vi "修改-微调探头测量值-30.vi"(8 "VI引用句柄":refnum<vi>, 10 "探头地址":i32, 11 "VISA资源名称":refnum<visa-resource-name>) -> (0 "结果":T1)   [LabVIEW 2017]
panel:
  in  "取消按钮":bool
  in  "确定按钮":bool
  in  "微调方向":enum8{"减小", "增大"}(ring)
  in  "微调值 uSv/h":sgl=0.03 min=0 max=655.36 format="%#.2f"
  out "提示语":string
  # "提示：微调值直接修改探头硬件参数，\n软件中无修改记录，请谨慎修改"
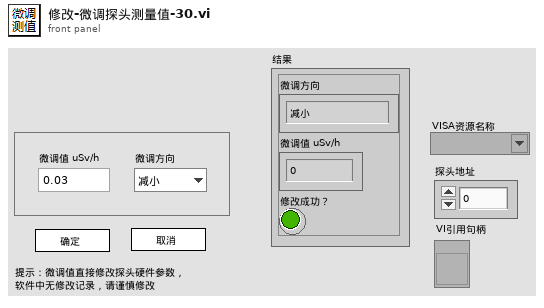
[diagram p1: front panel]
types:
  T1 = cluster{"微调方向":enum8{"减小", "增大"}, "微调值 uSv/h":sgl, "修改成功？":bool}
  T2 = enum32{"Invalid", "Standard", "Closed", "Hidden", "Minimized", "Maximized"}
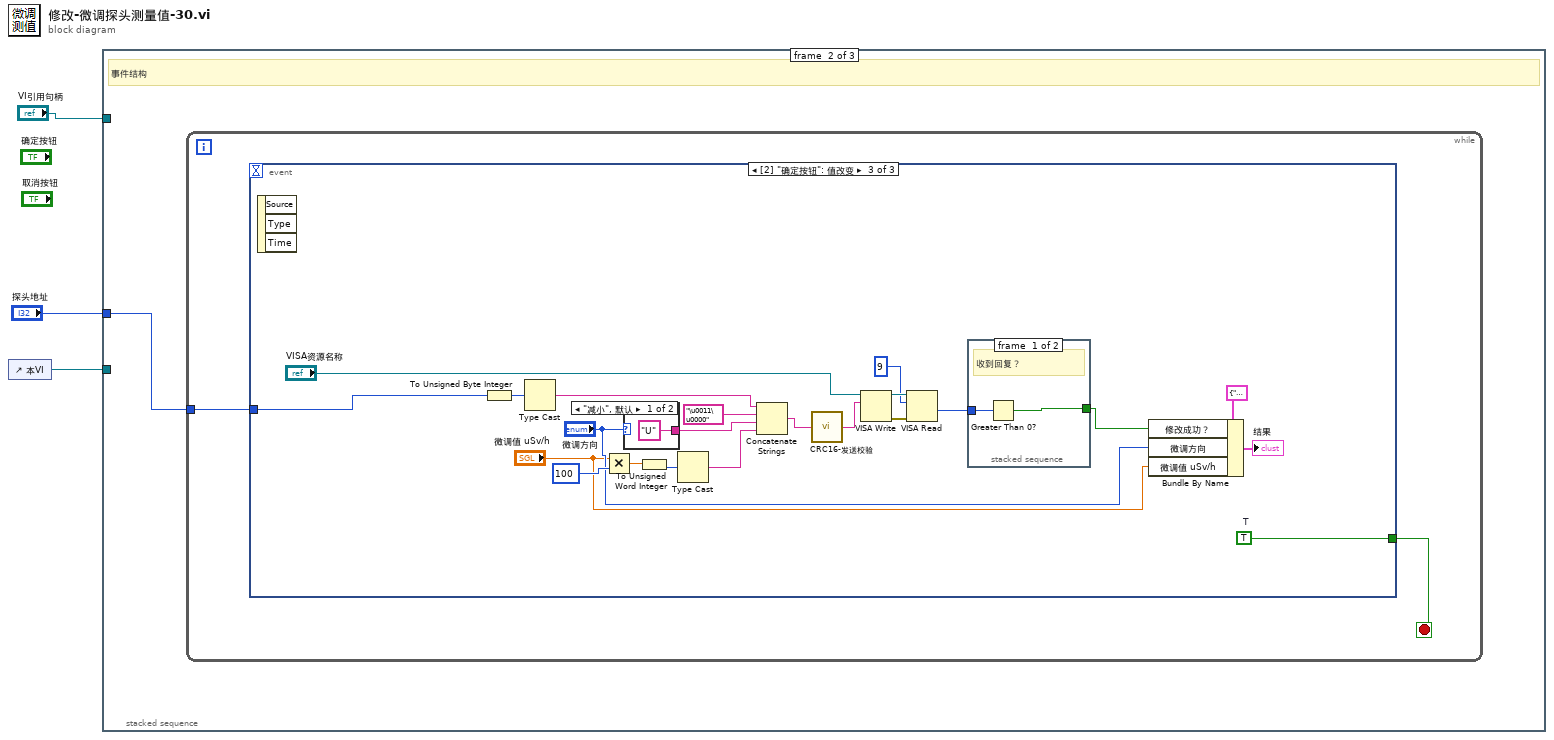
[diagram p0: block diagram]
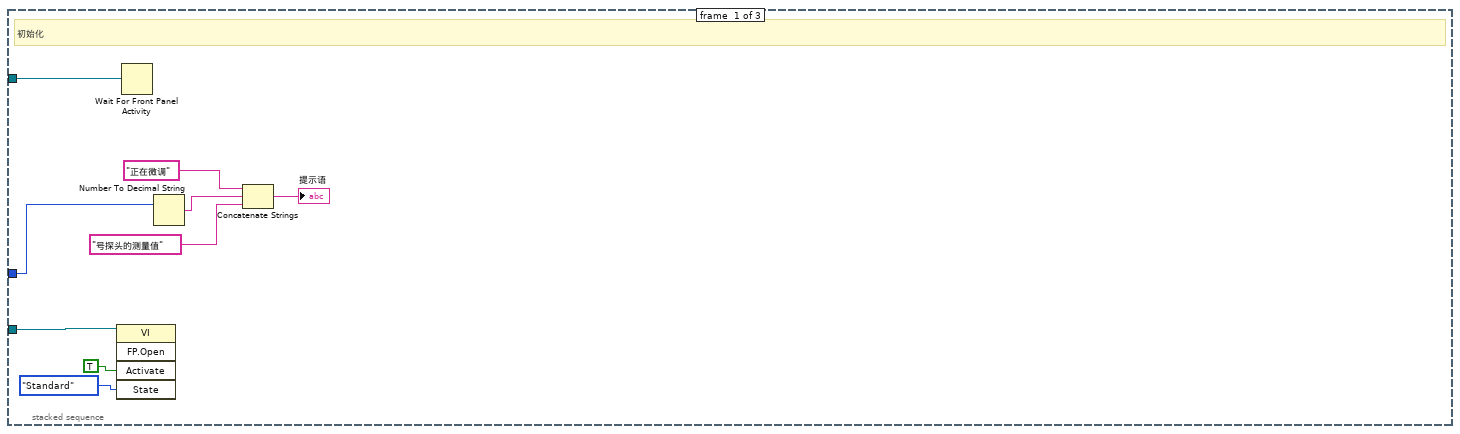
[diagram p2: hidden frame]
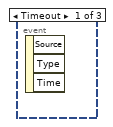
[diagram p3: hidden frame]
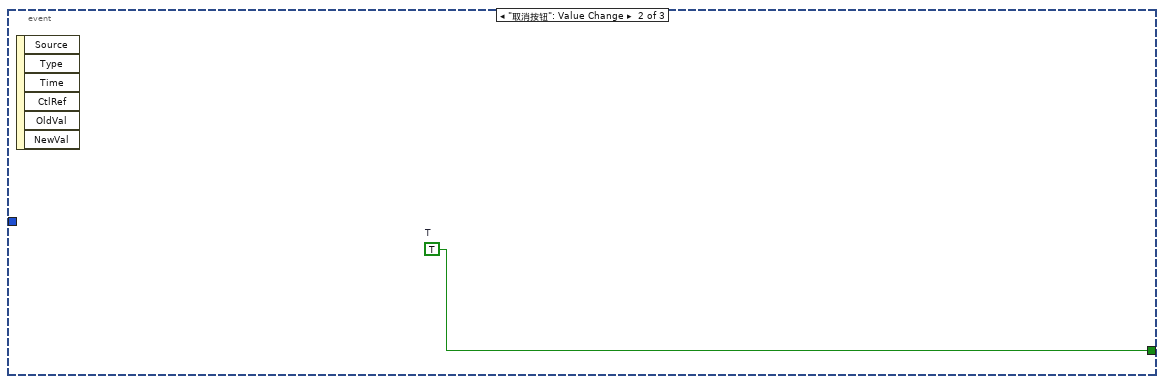
[diagram p4: hidden frame]
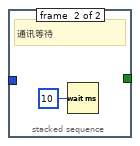
[diagram p5: hidden frame]
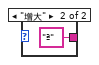
[diagram p6: hidden frame]
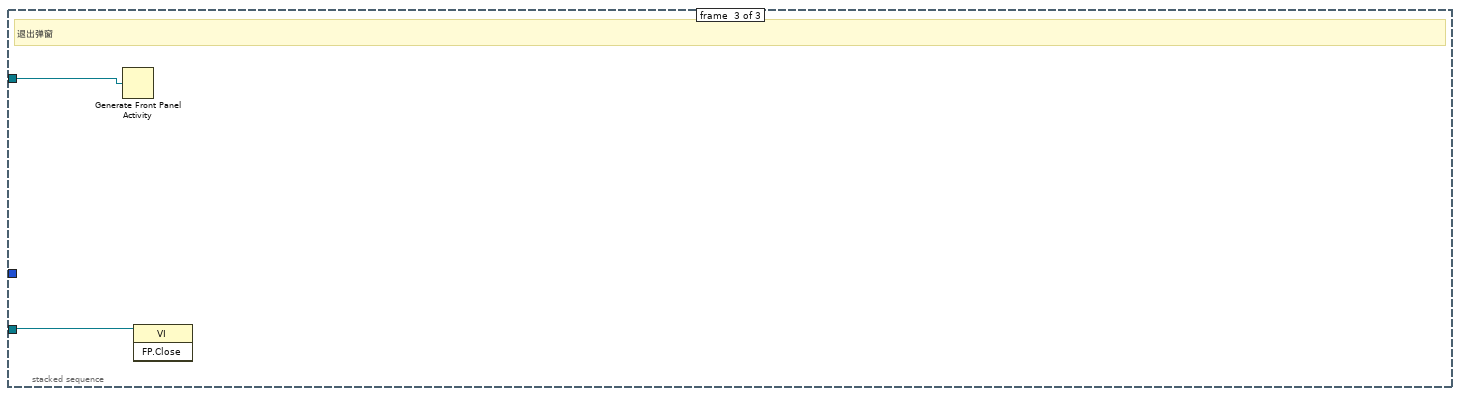
[diagram p7: hidden frame]
diagram:
  n1 = control-ref of="本VI"() -> (w1:refnum<vi>)
  n2 = stacked-sequence {
    tunnel: "VI引用句柄" -> [w8 _ w45]
    tunnel: "探头地址" -> [w7 w13 _]
    tunnel: w1 -> [w6 _ w44]
    frame #0 {
      # "初始化"
      n3 = invoke class="VI" method="FP.Open"(reference=w6, "Activate"=TRUE ("激活？"), "State"=T2."Standard" ("状态")) -> ()  [unwired: 2 in, 5 out]
      n4 = Wait For Front Panel Activity(2:w8) -> ()  [unwired: 2 in, 1 out]
      n5 = Number To Decimal String(number=w7) -> (decimal integer string=w11:string)  [unwired: 1 in]
      n6 = Concatenate Strings("正在微调" ("字符串"), w11, "号探头的测量值" ("字符串")) -> (→"提示语":string)
    }
    frame #1 {
      # "事件结构"
      n7 = while {
        tunnel: w13 -> [w14]
        stop <- w15 stop-if-true
        n8 = event shown="[2] \"确定按钮\": 值改变" {
          selector: _ -> [_ _ _]
          dyn-events: _ -> [_ _ _]
          timeout: _ -> [_ _ _]
          tunnel: [_ w16 w37] -> w15
          tunnel: w14 -> [_ _ w38]
          event Timeout {
            n9 = event-data() -> ()  [unwired: 1 in, 3 out]
          }
          event "取消按钮": Value Change {
            w16 = TRUE  # T
            n10 = event-data() -> ()  [unwired: 1 in, 6 out]
          }
          event "确定按钮": Value Change {
            w37 = TRUE  # T
            n11 = event-data() -> ()  [unwired: 1 in, 3 out]
            n12 = To Unsigned Byte Integer(number=w38) -> (unsigned 8bit integer=w28:u8)
            n13 = Type Cast(x=w28) -> (*(type *) &x=w35:string)  [unwired: 1 in]
            n14 = Multiply(x="微调值 uSv/h", y=100) -> (x*y=w31:sgl)
            n15 = case shown="\"减小\", 默认" "微调方向" {
              tunnel: ["U" "ª"] -> w33
              frame "减小", Default {
              }
              frame "增大" {
              }
            }
            n16 = To Unsigned Word Integer(number=w31) -> (unsigned 16bit integer=w32:u16)
            n17 = Type Cast(x=w32) -> (*(type *) &x=w34:string)  [unwired: 1 in]
            n18 = Concatenate Strings(w35, "\u0011\u0000", w33, w34) -> (w18:string)
            n19 = call "CRC16-发送校验.vi"("净数据"=w18) -> ("完整输出"=w17:string)
            n20 = VISA Write(VISA resource name="VISA资源名称", write buffer=w17) -> (VISA resource name out=w26:refnum<visa-resource-name>, error out=w27:errorcluster)  [unwired: 1 in, 1 out]
            n21 = VISA Read(VISA resource name=w26, byte count=u32 9 ("字节总数"), error in (no error)=w27) -> (return count=w25:u32)  [unwired: 3 out]
            n22 = stacked-sequence {
              tunnel: w25 -> [w40 _]
              tunnel: [w39 _] -> w22
              frame #0 {
                # "收到回复？"
                n23 = Greater Than 0?(x=w40) -> (x > 0?=w39:bool)
              }
              frame #1 {
                # "通讯等待"
                n24 = Wait (ms)(milliseconds to wait=u32 10 ("等待时间（毫秒）")) -> ()  [unwired: 1 out]
              }
            }
            n25 = Bundle By Name(cluster=T1 {"微调方向"=enum."减小", "微调值 uSv/h"=0.03, "修改成功？"=FALSE}, "修改成功？"=w22, "微调方向"="微调方向", "微调值 uSv/h"="微调值 uSv/h") -> (→"结果":T1)
          }
        }
      }
    }
    frame #2 {
      # "退出弹窗"
      n26 = Generate Front Panel Activity(w45) -> ()
      n27 = invoke class="VI" method="FP.Close"(reference=w44) -> ()  [unwired: 2 in, 3 out]
    }
  }
